vi "add ch.vi"(7 "tem":enum16{"Single-Ended", "Differential"}(ring), 9 "output cluster":T1, 11 "DAQmx Device Name OUT":tag) -> (1 "input cluster":T1)   [LabVIEW 2011]
uses:
  C:/Program Files/National Instruments/LabVIEW 8.6/resource/objmgr/daqmx.rc
  filter.ctl
  Power_config.ctl
  signal type.ctl
  gain.ctl
  single chanel.ctl
  CARD config.ctl
panel:
  out "Array":bool[](array[boolean])
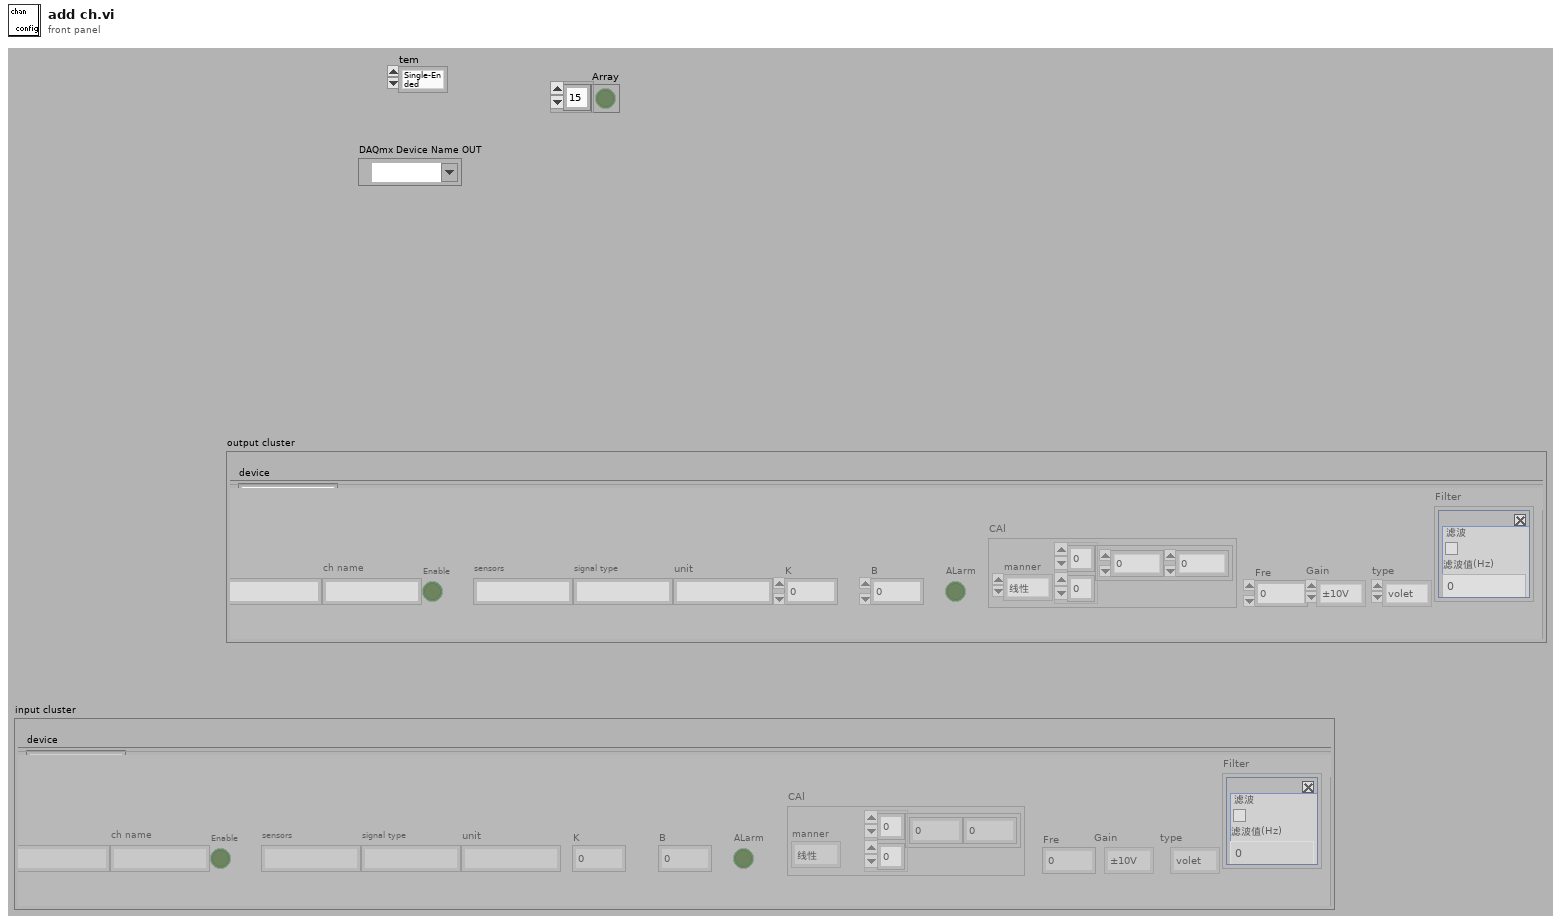
[diagram p1: front panel]
types:
  T1 = typedef "CARD config.ctl" = cluster{"device":string, "ch":T2[]}
  T2 = typedef "single chanel.ctl" = cluster{"chanel":string, "ch name":string, "Enable":bool, "sensors":string, "signal type":string, "unit":string, "K":dbl, "B":dbl, "ALarm":bool, "CAl":cluster{"manner":enum16{"线性", "查表"}, "data":dbl[][]}, "Fre":dbl, "type":T3, "Gain":T4, "Filter":T5, "Power":T6}
  T3 = typedef "signal type.ctl" = enum16{"未设置", "volet", "current", "vibration", "electric charge ", "resistance "}
  T4 = typedef "gain.ctl" = enum16{"±10V", "±5V", "±2.5V", "±1V", "±500mV", "±100mV", "10V", "5V", "2.5V", "1V", "500mV", "100mV"}
  T5 = typedef "filter.ctl" = cluster{"en":bool, "value":i32, "Boolean":bool}
  T6 = typedef "Power_config.ctl" = cluster{"power_en":bool, "Mode":enum16{"电压", "电流"}, "value":dbl, "Boolean":bool}
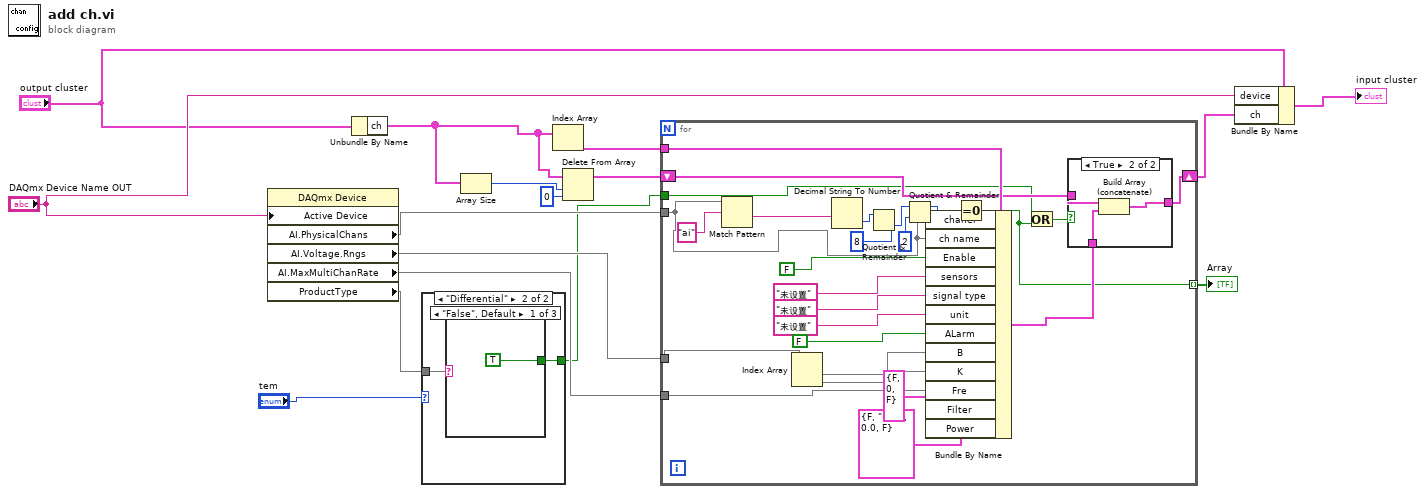
[diagram p0: block diagram]
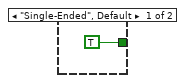
[diagram p2: hidden frame]
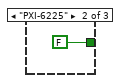
[diagram p3: hidden frame]
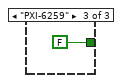
[diagram p4: hidden frame]
diagram:
  n1 = property class="DAQmx Device"("Active Device"="DAQmx Device Name OUT") -> ("AI.PhysicalChans"=w13, "AI.Voltage.Rngs"=w12, "AI.MaxMultiChanRate"=w11, "ProductType"=w4)  [unwired: 2 in, 2 out]
  n2 = Unbundle By Name("output cluster") -> ("ch"=w7:T2[])
  n3 = case shown="\"Differential\"" "tem" {
    tunnel: w4 -> [_ w19]
    tunnel: [TRUE w18] -> w3
    frame "Single-Ended", Default {
    }
    frame "Differential" {
      n4 = case shown="\"False\", Default" w19 {
        tunnel: [TRUE FALSE FALSE] -> w18
        frame "False", Default {
        }
        frame "PXI-6225" {
        }
        frame "PXI-6259" {
        }
      }
    }
  }
  n5 = Array Size(array=w7) -> (size(s)=w6:i32)
  n6 = Index Array(array=w7) -> (element=w15:T2)  [unwired: 1 in]
  n7 = Delete From Array(array=w7, length=w6, index=0) -> (array with subset deleted=w5:T2[])  [unwired: 1 out]
  n8 = for {
    tunnel: w15 -> [w43]
    tunnel: w13 -> [w37]
    tunnel: w12 -> [w41]
    tunnel: w11 -> [w42]
    shift-right: [w33] -> w16
    shift-left: w5 -> [w35]
    tunnel: w3 -> [w30]
    tunnel: [w26] -> w1 mode=indexing
    n9 = Match Pattern(string=w37, regular expression="ai") -> (after substring=w28:string)  [unwired: 4 out]
    n10 = Index Array(array=w41) -> (element #1=w40, element #2=w39)  [unwired: 2 in]
    n11 = Decimal String To Number(string=w28) -> (number=w27:i32)  [unwired: 3 out]
    n12 = Quotient & Remainder(x=w27, y=8) -> (floor(x/y)=w32:i32)  [unwired: 1 out]
    n13 = Quotient & Remainder(x=w32, y=2) -> (x-y*floor(x/y)=w25:i32)  [unwired: 1 out]
    n14 = Bundle By Name(cluster=w43, "chanel"=w37, "ch name"=w37, "Enable"=FALSE, "sensors"="未设置", "signal type"="未设置", "unit"="未设置", "ALarm"=FALSE, "B"=w40, "K"=w39, "Fre"=w42, "Filter"=T5 {"en"=FALSE, "value"=0, "Boolean"=FALSE}, "Power"=T6 {"power_en"=FALSE, "Mode"=enum."电压", "value"=0.0, "Boolean"=FALSE}) -> (w34:T2)
    n15 = Equal To 0?(x=w25) -> (x = 0?=w26:bool)
    n16 = Or(x=w30, y=w26) -> (x .or. y?=w29:bool)
    n17 = case shown="True" w29 {
      tunnel: w35 -> [w49 w52]
      tunnel: [w49 w51] -> w33
      tunnel: w34 -> [_ w50]
      frame False {
      }
      frame True {
        n18 = Build Array (concatenate)(w52, w50) -> (w51:T2[])
      }
    }
  }
  "Array" <- w1
  n19 = Bundle By Name(cluster="output cluster", "device"="DAQmx Device Name OUT", "ch"=w16) -> (→"input cluster":T1)
